vi "QueryStatus.vi"(8 "error in (no error)":errorcluster, 11 "RMX4120 in":refnum<class "RMX4120.lvclass">) -> (0 "error out":errorcluster, 1 "Error Message":string, 2 "Error Code":i32[](array[numeric]), 3 "RMX4120 out":refnum<class "RMX4120.lvclass">)   [LabVIEW 2023, in "RMX4120.lvclass"]
uses:
  RMX4120.lvclass
  RMXPowerSupply.lvclass
  RMX4120.lvclass/RMX4120.ctl
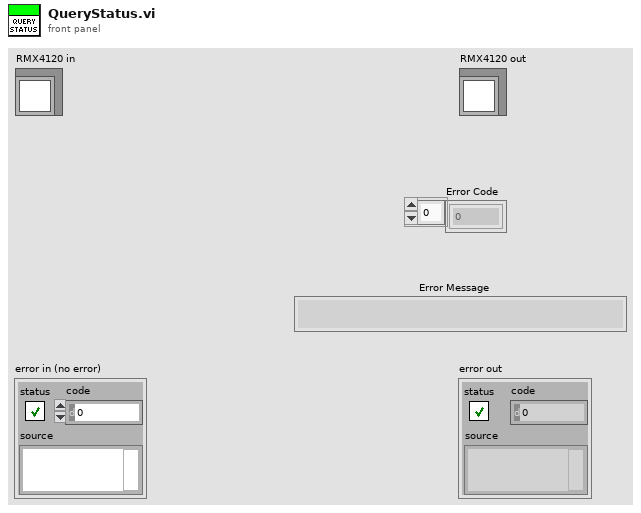
[diagram p1: front panel]
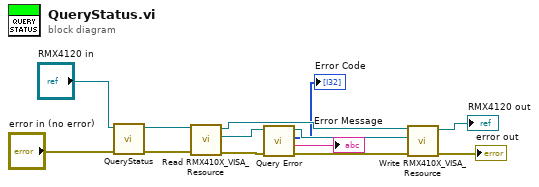
[diagram p0: block diagram]
diagram:
  n1 = call-parent "QueryStatus.vi"("error in (no error)"="error in (no error)", "RMXPowerSupply in"="RMX4120 in") -> ("error out"=w6:errorcluster, "RMXPowerSupply out"=w8:refnum<class "RMX4120.lvclass">)  [unwired: 6 in, 2 out]
  n2 = call-dynamic "Read RMX410X_VISA_Resource.vi"("error in (no error)"=w6, "RMXPowerSupply in"=w8) -> ("error out"=w10:errorcluster, "RMX410X_VISA_Resource"=w4:refnum<visa-resource-name>, "RMXPowerSupply out"=w11:refnum<class "RMX4120.lvclass">)  [unwired: 7 in]
  n3 = call "Query Error.vi"("error in (no error)"=w10, "VISA resource name"=w4) -> ("error out"=w9:errorcluster, "Error Message"=→"Error Message":string, "Error Code"=→"Error Code":i32[], "VISA resource name out"=w3:refnum<visa-resource-name>)  [unwired: 6 in]
  n4 = call-dynamic "Write RMX410X_VISA_Resource.vi"("error in (no error)"=w9, "RMX410X_VISA_Resource"=w3, "RMXPowerSupply in"=w11) -> ("error out"=→"error out":errorcluster, "RMXPowerSupply out"=→"RMX4120 out":refnum<class "RMX4120.lvclass">)  [unwired: 7 in]
